vi "Read T.vi"(11 "valve_VCH_ZM_state in":refnum<class "HE_ZM_state.lvclass">) -> (2 "T (ms)":u32, 3 "valve_VCH_ZM_state out":refnum<class "HE_ZM_state.lvclass">)   [LabVIEW 2019, in "Heating.lvlib" / "HE_ZM_state.lvclass"]
uses:
  HE_ZM_state.lvclass
  D:/my_projects/projects/Algorithms/Labview/19/Sequence/State/State.lvclass
  Sequence/State/State.lvclass/State.ctl
  Sequence/State/State.lvclass
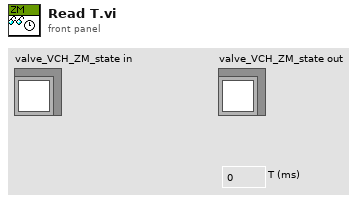
[diagram p1: front panel]
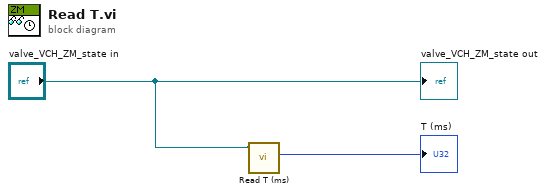
[diagram p0: block diagram]
diagram:
  n1 = call "Read T (ms).vi"("State in"="valve_VCH_ZM_state in") -> ("T (ms)"=→"T (ms)":u32)  [unwired: 9 in, 1 out]
  "valve_VCH_ZM_state out" <- "valve_VCH_ZM_state in"
